vi "GetBuildArguments.vi"() -> (0 "error out":errorcluster, 2 "output cluster":cluster{"Path ":path, string})   [LabVIEW 2020]
uses:
  <vilib>/Utility/error.llb/Error Cluster From Error Code.vi
  <vilib>/ErrorRing/Error Ring.xnode
panel:
  in  "error in":errorcluster
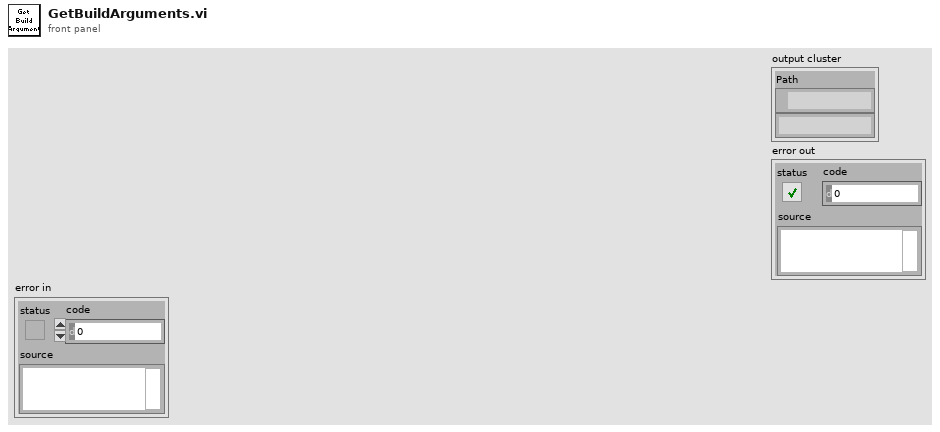
[diagram p1: front panel]
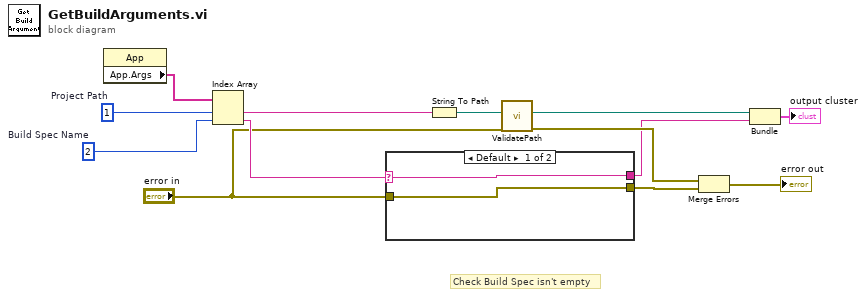
[diagram p0: block diagram]
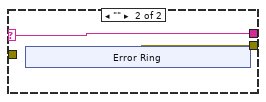
[diagram p2: hidden frame]
diagram:
  w10 = 2  # Build Spec Name
  w11 = 1  # Project Path
  # "Check Build Spec isn't empty"
  n1 = property class="App"() -> ("App.Args"=w13:string[])  [unwired: 2 in, 2 out]
  n2 = Index Array(array=w13, index #1=w11, index #2=w10) -> (element #1=w12:string, element #2=w8:string)
  n3 = case shown="Default" w8 {
    selector: w8 -> [w15 w17]
    tunnel: [w15 w17] -> w3
    tunnel: [w14 w16] -> w7
    tunnel: "error in" -> [w14 _]
    frame Default {
    }
    frame "" {
      n4 = xnode "Error Ring"() -> ("error out"=w16:errorcluster)
    }
  }
  n5 = String To Path(string=w12) -> (path=w9:path)
  n6 = call "ValidatePath.vi"("error constant"="error in", "Path"=w9) -> ("error inditcator 2"=w6:errorcluster, "Path"=w4:path)  [unwired: 8 in]
  n7 = Merge Errors(w6, w7) -> (→"error out":errorcluster)
  n8 = Bundle("Path"=w4, w3) -> (→"output cluster":cluster{"Path ":path, string})  [unwired: 1 in]
